vi "tb_Cascade Logic.vi"() -> ()   [LabVIEW 2011]
uses:
  <instrlib>/RF-RIO/Memory/FPGA/Interface/Retrieve Data (128-Bit).ctl
  <instrlib>/RF-RIO/Memory/FPGA/Interface/U128.ctl
  Data Type (256).ctl
  <instrlib>/RF-RIO/Memory/FPGA/Memory.lvlib
panel:
  out "Cascaded Bank Status":T1
  out "Output Data":T2
  out "Output Valid":bool
  in  "Bank0 Data":T3
  in  "Bank0 Status":T5
  in  "Bank1 Data":T3
  in  "Bank1 Status":T5
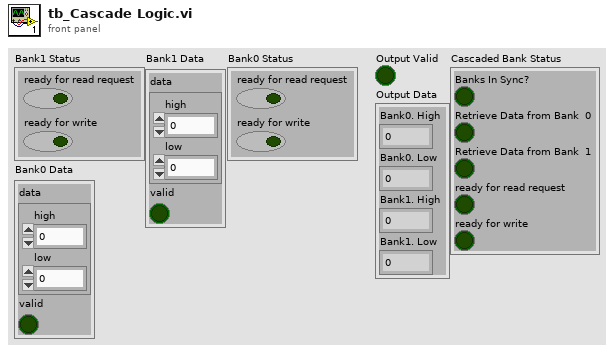
[diagram p1: front panel]
types:
  T1 = cluster{"Banks In Sync?":bool, "Retrieve Data from Bank  0":bool, "Retrieve Data from Bank  1":bool, "ready for read request":bool, "ready for write":bool}
  T2 = typedef "Data Type (256).ctl" = cluster{"Bank0. High":u64, "Bank0. Low":u64, "Bank1. High":u64, "Bank1. Low":u64}
  T3 = typedef "Memory.lvlib/Retrieve Data (128-Bit).ctl" = cluster{"data":T4, "valid":bool}
  T4 = typedef "Memory.lvlib/U128.ctl" = cluster{"high":u64, "low":u64}
  T5 = cluster{"ready for read request":bool, "ready for write":bool}
  T6 = typedef "Cascaded Bank Status.ctl" = cluster{"Banks In Sync?":bool, "RetrieveData from Bank  0":bool, "RetrieveData from Bank  1":bool, "ready for read request":bool, "ready for write":bool}
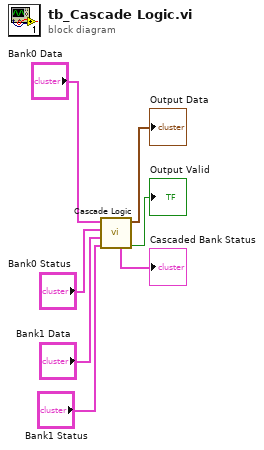
[diagram p0: block diagram]
diagram:
  n1 = call "Cascade Logic.vi"("Bank1 Status"="Bank1 Status", "Bank1 Data"="Bank1 Data", "Bank0 Status"="Bank0 Status", "Bank0 Data"="Bank0 Data") -> ("Output Valid"=→"Output Valid":bool, "Output Data"=→"Output Data":T2, "Cascaded Bank Status"=→"Cascaded Bank Status":T6)  [unwired: 5 in]
